vi "LVIS_InitGlobals.vi"(8 "Error In":errorcluster) -> (0 "Error Out":errorcluster)   [LabVIEW 2015]
doc: "Initializes the global variables that will be used throughout the LVIS Library."
uses:
  Ctrls/LVIS_Msg State.ctl
  Globals/LVIS_IsGlobal.vi
  Globals/LVIS_DcGlobals.vi
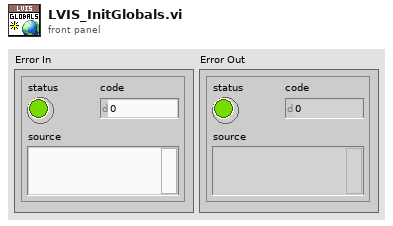
[diagram p1: front panel]
types:
  T1 = cluster{"EventName":string, "EventStart":string, "EventStop":string, "EventStatus":string, "EventClientID":string, "IS_EventID":string, "EventMeta":string, "ProductLine":string, "ProcessName":string, "Station":string, "Operator":string, "SN":string, "Model":string, "Manufacturer":string}
  T2 = typedef "LVIS_Msg State.ctl" = enum16{"None", "Offline", "Online", "Backup Full"}
  T3 = cluster{"EventInfo":cluster{"EventName":string, "EventStart":string, "EventStop":string, "EventStatus":string, "EventClientID":string, "IS_EventID":string, "EventMeta":string, "ProductLine":string, "ProcessName":string, "Station":string, "Operator":string, "SN":string, "Model":string, "Manufacturer":string}, "TestInfo":cluster{"TestName":string, "TestDateTime":string, "TestStatus":string, "TestClientID":string, "IS_TestID":string, "TestMeta":string}, "MeasInfo":cluster{"MeasName":string, "MeasDateTime":string, "MeasStatus":string, "MeasClientID":string, "IS_MeasID":string, "MeasType":string, "MeasValue":string, "LL":string, "LL Comp":string, "HL":string, "HL Comp":string, "Units":string, "MeasMeta":string}}[]
  T4 = cluster{"MeasName":string, "MeasDateTime":string, "MeasStatus":string, "MeasClientID":string, "IS_MeasID":string, "MeasType":string, "MeasValue":string, "LL":string, "LL Comp":string, "HL":string, "HL Comp":string, "Units":string, "MeasMeta":string}
  T5 = cluster{"TestName":string, "TestDateTime":string, "TestStatus":string, "TestClientID":string, "IS_TestID":string, "TestMeta":string}
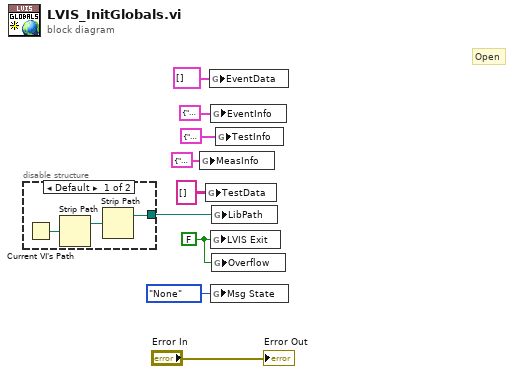
[diagram p0: block diagram]
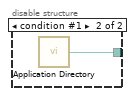
[diagram p2: hidden frame]
diagram:
  w3 = FALSE ("LVIS Exit")
  # "Open"
  n1 = disable-structure shown="Default" {
    disable-tunnel: [w10 w13] -> w1
    frame condition #0 (active) {
      n2 = Current VI's Path() -> (path=w11:path)
      n3 = Strip Path(path=w11) -> (stripped path=w12:path)  [unwired: 1 out]
      n4 = Strip Path(path=w12) -> (stripped path=w10:path)  [unwired: 1 out]
    }
    frame condition #1 {
      n5 = call <vilib>:"Application Directory.vi"() -> ("Application Directory"=w13:path)
    }
  }
  n6 = global write "LVIS_IsGlobal.vi" "MeasInfo"(T4 {"MeasName"="", "MeasDateTime"="", "MeasStatus"="", "MeasClientID"="", "IS_MeasID"="", "MeasType"="", "MeasValue"="", "LL"="", "LL Comp"="", "HL"="", "HL Comp"="", "Units"="", "MeasMeta"=""} ("MeasInfo")) -> ()
  n7 = global write "LVIS_IsGlobal.vi" "TestData"(string[][][] [] ("TestData")) -> ()
  n8 = global write "LVIS_IsGlobal.vi" "EventData"(T3 [] ("EventData")) -> ()
  n9 = global write "LVIS_IsGlobal.vi" "EventInfo"(T1 {"EventName"="*", "EventStart"="*", "EventStop"="*", "EventStatus"="*", "EventClientID"="*", "IS_EventID"="*", "EventMeta"="", "ProductLine"="*", "ProcessName"="*", "Station"="*", "Operator"="*", "SN"="*", "Model"="*", "Manufacturer"="*"} ("EventInfo")) -> ()
  n10 = global write "LVIS_DcGlobals.vi" "LVIS Exit"(w3) -> ()
  n11 = global write "LVIS_DcGlobals.vi" "Msg State"(LVIS_Msg_State."None" ("Msg State")) -> ()
  n12 = global write "LVIS_IsGlobal.vi" "LibPath"(w1) -> ()
  n13 = global write "LVIS_DcGlobals.vi" "Overflow"(w3) -> ()
  n14 = global write "LVIS_IsGlobal.vi" "TestInfo"(T5 {"TestName"="", "TestDateTime"="", "TestStatus"="", "TestClientID"="", "IS_TestID"="", "TestMeta"=""} ("TestInfo")) -> ()
  "Error Out" <- "Error In"
